vi "_Main.vi"   [LabVIEW 2017, in "Hopper System.lvlib"]
uses:
  Hopper System.lvlib
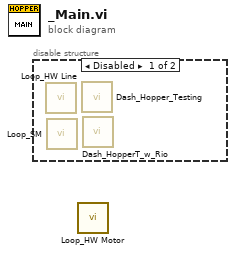
[diagram p0: block diagram]
diagram:
  n1 = disable-structure shown="Disabled" {
    frame Disabled {
      n2 = call "Loop_HW Line.vi"() -> ()  [unwired: 12 in]
      n3 = call "Loop_SM.vi"() -> ()  [unwired: 12 in]
      n4 = call "Dash_Hopper_Testing.vi"() -> ()  [unwired: 12 in]
      n5 = call "Dash_HopperT_w_Rio.vi"() -> ()  [unwired: 12 in]
    }
    frame Enabled {
    }
  }
  n6 = call "Loop_HW Motor.vi"() -> ()  [unwired: 12 in]
